vi "Init PV-State.vi"(8 "error in (no error)":errorcluster, 11 "CS++Motor in":refnum<class "CS++Motor.lvclass">) -> (0 "error out":errorcluster, 3 "CS++Motor out":refnum<class "CS++Motor.lvclass">)   [LabVIEW 2015, in "CS++Motor.lvlib" / "CS++Motor.lvclass"]
doc: "this VI helps with the initialization of the variables needed in the Actor Core."
uses:
  CS++Motor.lvclass
  CSPP_Core/Classes/CS++ProcessVariables/ProcessVariable/PV.lvclass
  CS++Motor.lvclass/CS++Motor.ctl
  CSPP_Core/Classes/CS++ProcessVariables/ProcessVariable/PV.lvclass/PV.ctl
  CSPP_Core/Classes/CS++ProcessVariables/ProcessVariable/Write PV URL.vi
  CSPP_Core/Classes/CS++ProcessVariables/ProcessVariable/Write Type Descriptor.vi
  <vilib>/Utility/error.llb/Error Cluster From Error Code.vi
  CSPP_Core/Classes/CS++ProcessVariables/PVConnection/PVConnection.lvclass
  CSPP_Core/Classes/CS++ProcessVariables/CS++ProcessVariables.lvlib
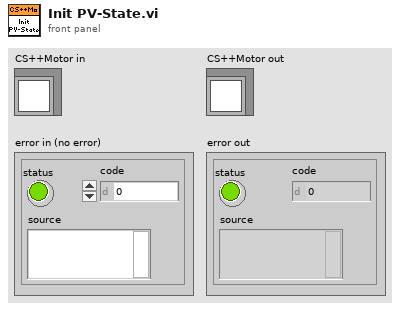
[diagram p1: front panel]
types:
  T1 = cluster{"LogicalName":string, "PhysicalName":string, "unit":string, "Scaling":dbl, "Scaling Offset":dbl, "StartVelocity":dbl, "StopVelocity":dbl, "Acceleration":dbl, "RangeMin":dbl, "RangeMax":dbl, "LogicalPos-Array":cluster{"LogicalPosition":string, "SetPosition":dbl}[]}[]
  T2 = cluster{"RawActPosition":string[], "Referenced":string[], "Error":string[], "Moving":string[]}
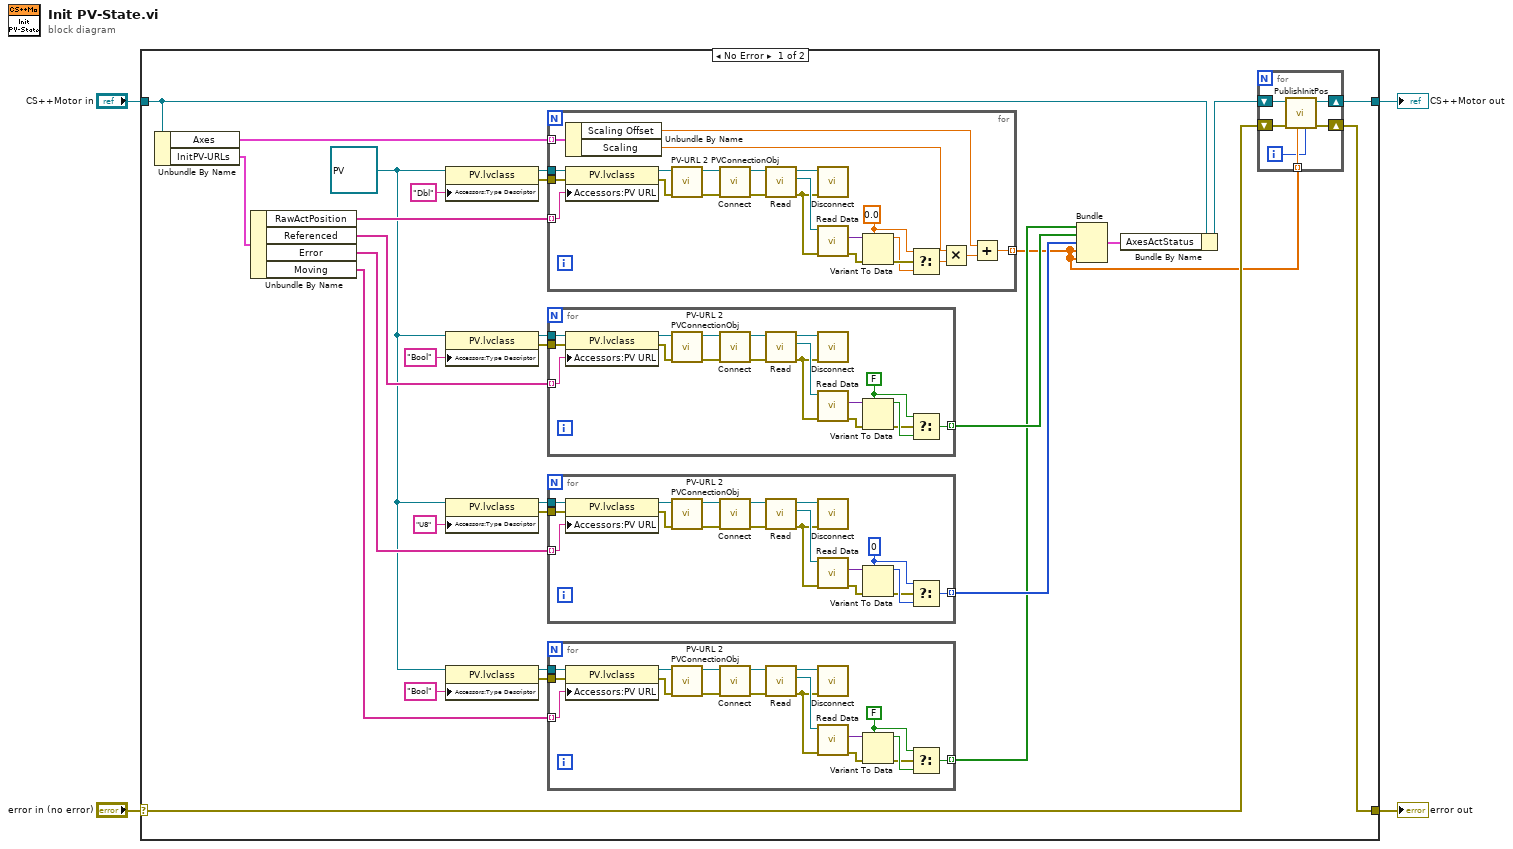
[diagram p0: block diagram]
diagram:
  n1 = case shown="No Error" "error in (no error)" {
    selector: "error in (no error)" -> [w7 w118]
    tunnel: [w6 w118] -> w3
    tunnel: [w8 w117] -> w2
    tunnel: "CS++Motor in" -> [w11 w117]
    frame No Error {
      w13 = refnum<class "PV.lvclass"> refnum ("CS++ProcessVariables.lvlib:PV.lvclass")
      n2 = Unbundle By Name(w11) -> ("Axes"=w24:T1, "InitPV-URLs"=w33:T2)
      n3 = Unbundle By Name(w33) -> ("RawActPosition"=w29:string[], "Referenced"=w25:string[], "Error"=w19:string[], "Moving"=w14:string[])
      n4 = property class="PV.lvclass"(reference=w13, "Accessors:Type Descriptor"="Dbl" ("Type Descriptor")) -> (reference out=w32:refnum<class "PV.lvclass">, error out=w31:errorcluster)  [unwired: 1 in]
      n5 = property class="PV.lvclass"(reference=w13, "Accessors:Type Descriptor"="Bool" ("Type Descriptor")) -> (reference out=w26:refnum<class "PV.lvclass">, error out=w27:errorcluster)  [unwired: 1 in]
      n6 = property class="PV.lvclass"(reference=w13, "Accessors:Type Descriptor"="U8" ("Type Descriptor")) -> (reference out=w22:refnum<class "PV.lvclass">, error out=w21:errorcluster)  [unwired: 1 in]
      n7 = property class="PV.lvclass"(reference=w13, "Accessors:Type Descriptor"="Bool" ("Type Descriptor")) -> (reference out=w15:refnum<class "PV.lvclass">, error out=w16:errorcluster)  [unwired: 1 in]
      n8 = for {
        tunnel: w32 -> [w114]
        tunnel: w31 -> [w113]
        tunnel: w29 -> [w105] mode=indexing
        tunnel: w24 -> [w103] mode=indexing
        tunnel: [w97] -> w5 mode=indexing
        w99 = 0.0
        n9 = Unbundle By Name(w103) -> ("Scaling Offset"=w96:dbl, "Scaling"=w94:dbl)
        n10 = property class="PV.lvclass"(reference=w114, error in=w113, "Accessors:PV URL"=w105) -> (reference out=w116:refnum<class "PV.lvclass">, error out=w115:errorcluster)
        n11 = call "PV-URL 2 PVConnectionObj.vi"("Error In"=w115, "PV"=w116) -> ("Error Out"=w108:errorcluster, "PVConnection"=w109:refnum<class "PVConnection.lvclass">)  [unwired: 7 in, 1 out]
        n12 = call "Connect.vi"("Error In"=w108, "PVConnection in"=w109) -> ("Error Out"=w110:errorcluster, "PVConnection out"=w112:refnum<class "PVConnection.lvclass">)  [unwired: 8 in]
        n13 = call "Read.vi"("error in (no error)"=w110, "PVConnection in"=w112) -> ("error out"=w100:errorcluster, "PV"=w107:refnum<class "PV.lvclass">, "PVConnection out"=w111:refnum<class "PVConnection.lvclass">)  [unwired: 6 in, 1 out]
        n14 = call "Disconnect.vi"("error in (no error)"=w100, "PVConnection in"=w111) -> ()  [unwired: 8 in, 2 out]
        n15 = call "Read Data.vi"("error in (no error)"=w100, "PV in"=w107) -> ("error out"=w101:errorcluster, "Data"=w106:variant)  [unwired: 7 in, 1 out]
        n16 = Variant To Data(error in=w101, type=w99, Variant=w106) -> (data=w102:dbl, error out=w104:errorcluster)
        n17 = Select(t=w99, s=w104, f=w102) -> (s? t:f=w98:dbl)
        n18 = Multiply(x=w94, y=w98) -> (x*y=w95:dbl)
        n19 = Add(x=w96, y=w95) -> (x+y=w97:dbl)
      }
      n20 = for {
        tunnel: w26 -> [w91]
        tunnel: w27 -> [w90]
        tunnel: w25 -> [w82] mode=indexing
        tunnel: [w78] -> w23 mode=indexing
        w76 = FALSE
        n21 = property class="PV.lvclass"(reference=w91, error in=w90, "Accessors:PV URL"=w82) -> (reference out=w93:refnum<class "PV.lvclass">, error out=w92:errorcluster)
        n22 = call "PV-URL 2 PVConnectionObj.vi"("Error In"=w92, "PV"=w93) -> ("Error Out"=w85:errorcluster, "PVConnection"=w86:refnum<class "PVConnection.lvclass">)  [unwired: 7 in, 1 out]
        n23 = call "Connect.vi"("Error In"=w85, "PVConnection in"=w86) -> ("Error Out"=w87:errorcluster, "PVConnection out"=w89:refnum<class "PVConnection.lvclass">)  [unwired: 8 in]
        n24 = call "Read.vi"("error in (no error)"=w87, "PVConnection in"=w89) -> ("error out"=w79:errorcluster, "PV"=w84:refnum<class "PV.lvclass">, "PVConnection out"=w88:refnum<class "PVConnection.lvclass">)  [unwired: 6 in, 1 out]
        n25 = call "Disconnect.vi"("error in (no error)"=w79, "PVConnection in"=w88) -> ()  [unwired: 8 in, 2 out]
        n26 = call "Read Data.vi"("error in (no error)"=w79, "PV in"=w84) -> ("error out"=w80:errorcluster, "Data"=w83:variant)  [unwired: 7 in, 1 out]
        n27 = Variant To Data(error in=w80, type=w76, Variant=w83) -> (data=w81:bool, error out=w77:errorcluster)
        n28 = Select(t=w76, s=w77, f=w81) -> (s? t:f=w78:bool)
      }
      n29 = for {
        tunnel: w22 -> [w73]
        tunnel: w21 -> [w72]
        tunnel: w19 -> [w64] mode=indexing
        tunnel: [w60] -> w18 mode=indexing
        w58 = u8 0
        n30 = property class="PV.lvclass"(reference=w73, error in=w72, "Accessors:PV URL"=w64) -> (reference out=w75:refnum<class "PV.lvclass">, error out=w74:errorcluster)
        n31 = call "PV-URL 2 PVConnectionObj.vi"("Error In"=w74, "PV"=w75) -> ("Error Out"=w67:errorcluster, "PVConnection"=w68:refnum<class "PVConnection.lvclass">)  [unwired: 7 in, 1 out]
        n32 = call "Connect.vi"("Error In"=w67, "PVConnection in"=w68) -> ("Error Out"=w69:errorcluster, "PVConnection out"=w71:refnum<class "PVConnection.lvclass">)  [unwired: 8 in]
        n33 = call "Read.vi"("error in (no error)"=w69, "PVConnection in"=w71) -> ("error out"=w61:errorcluster, "PV"=w66:refnum<class "PV.lvclass">, "PVConnection out"=w70:refnum<class "PVConnection.lvclass">)  [unwired: 6 in, 1 out]
        n34 = call "Disconnect.vi"("error in (no error)"=w61, "PVConnection in"=w70) -> ()  [unwired: 8 in, 2 out]
        n35 = call "Read Data.vi"("error in (no error)"=w61, "PV in"=w66) -> ("error out"=w62:errorcluster, "Data"=w65:variant)  [unwired: 7 in, 1 out]
        n36 = Variant To Data(error in=w62, type=w58, Variant=w65) -> (data=w63:u8, error out=w59:errorcluster)
        n37 = Select(t=w58, s=w59, f=w63) -> (s? t:f=w60:u8)
      }
      n38 = for {
        tunnel: w15 -> [w55]
        tunnel: w16 -> [w54]
        tunnel: w14 -> [w46] mode=indexing
        tunnel: [w42] -> w12 mode=indexing
        w40 = FALSE
        n39 = property class="PV.lvclass"(reference=w55, error in=w54, "Accessors:PV URL"=w46) -> (reference out=w57:refnum<class "PV.lvclass">, error out=w56:errorcluster)
        n40 = call "PV-URL 2 PVConnectionObj.vi"("Error In"=w56, "PV"=w57) -> ("Error Out"=w49:errorcluster, "PVConnection"=w50:refnum<class "PVConnection.lvclass">)  [unwired: 7 in, 1 out]
        n41 = call "Connect.vi"("Error In"=w49, "PVConnection in"=w50) -> ("Error Out"=w51:errorcluster, "PVConnection out"=w53:refnum<class "PVConnection.lvclass">)  [unwired: 8 in]
        n42 = call "Read.vi"("error in (no error)"=w51, "PVConnection in"=w53) -> ("error out"=w43:errorcluster, "PV"=w48:refnum<class "PV.lvclass">, "PVConnection out"=w52:refnum<class "PVConnection.lvclass">)  [unwired: 6 in, 1 out]
        n43 = call "Disconnect.vi"("error in (no error)"=w43, "PVConnection in"=w52) -> ()  [unwired: 8 in, 2 out]
        n44 = call "Read Data.vi"("error in (no error)"=w43, "PV in"=w48) -> ("error out"=w44:errorcluster, "Data"=w47:variant)  [unwired: 7 in, 1 out]
        n45 = Variant To Data(error in=w44, type=w40, Variant=w47) -> (data=w45:bool, error out=w41:errorcluster)
        n46 = Select(t=w40, s=w41, f=w45) -> (s? t:f=w42:bool)
      }
      n47 = Bundle(w12, w23, w18, w5, w5) -> (w10:cluster{bool[], bool[], u8[], dbl[], dbl[]})  [unwired: 1 in]
      n48 = Bundle By Name(cluster=w11, "AxesActStatus"=w10) -> (w9:refnum<class "CS++Motor.lvclass">)
      n49 = for {
        shift-right: [w38] -> w8
        shift-left: w9 -> [w39]
        shift-right: [w36] -> w6
        shift-left: w7 -> [w37]
        tunnel: w5 -> [w35] mode=indexing
        i -> [w34]
        n50 = call "PublishInitPos.vi"("AxisNumber"=w34, "ActPos"=w35, "error in (no error)"=w37, "CS++Motor in"=w39) -> ("error out"=w36:errorcluster, "CS++Motor out"=w38:refnum<class "CS++Motor.lvclass">)  [unwired: 6 in]
      }
    }
    frame Error {
    }
  }
  "error out" <- w3
  "CS++Motor out" <- w2
